vi "PicoScope6000ClearStreming.vi"(8 "error in (no error)":errorcluster, 11 "handle":i16) -> (0 "error out":errorcluster, 3 "handle out":i16)   [LabVIEW 2009]
doc: "This closes the oscilloscope and should be called before exiting an application."
uses:
  ps6000Wrap.dll
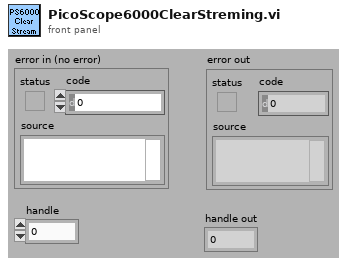
[diagram p1: front panel]
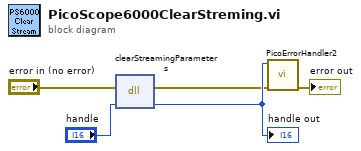
[diagram p0: block diagram]
diagram:
  n1 = dll-call lib="ps6000Wrap.dll" fn="clearStreamingParameters"(error in="error in (no error)", "handle"="handle") -> (error out=w1:errorcluster, "handle"=w2:i16)  [unwired: 3 in, 1 out]
  "handle out" <- w2
  n2 = call "PicoErrorHandler2.vi"("error in (no error)"=w1, "handle In"=w2) -> ("error out"=→"error out":errorcluster)  [unwired: 9 in]
